vi "fmt_formatDataColumn.vi"(5 "styles map":string[](array[string]), 8 "error in (no error)":errorcluster, 9 "data":T1, 10 "channel index":i32, 11 "Format buffers in":T3) -> (0 "error out":errorcluster, 3 "Format buffers out":T3)   [LabVIEW 2017, in "NI_ExcelFile.lvlib"]
uses:
  <vilib>/express/express shared/NI_ExcelFile/NI_ExcelFile.lvlib
  <vilib>/express/express shared/NI_ExcelFile/Ctrls/fmt_formatBuffer.ctl
  <vilib>/express/express shared/NI_ExcelFile/Ctrls/TimeColumnMode.ctl
  <vilib>/express/express shared/NI_ExcelFile/Ctrls/Columns.ctl
  <vilib>/express/express shared/NI_ExcelFile/Ctrls/ColumnInfo.ctl
  <vilib>/express/express shared/NI_ExcelFile/Ctrls/DataType.ctl
  <vilib>/express/express shared/NI_ExcelFile/Ctrls/data_AllTypeData.ctl
  <vilib>/express/express shared/NI_ExcelFile/SubVIs/fmt_formatSingleCell (Numeric).vi
  <vilib>/express/express shared/NI_ExcelFile/SubVIs/fmt_timestampToExcel.vi
  <vilib>/express/express shared/NI_ExcelFile/SubVIs/fmt_formatSingleCell (String).vi
  <vilib>/express/express shared/NI_ExcelFile/SubVIs/fmt_escapeXML.vi
  <vilib>/express/express shared/NI_ExcelFile/SubVIs/fmt_getUTF-8Text.vi
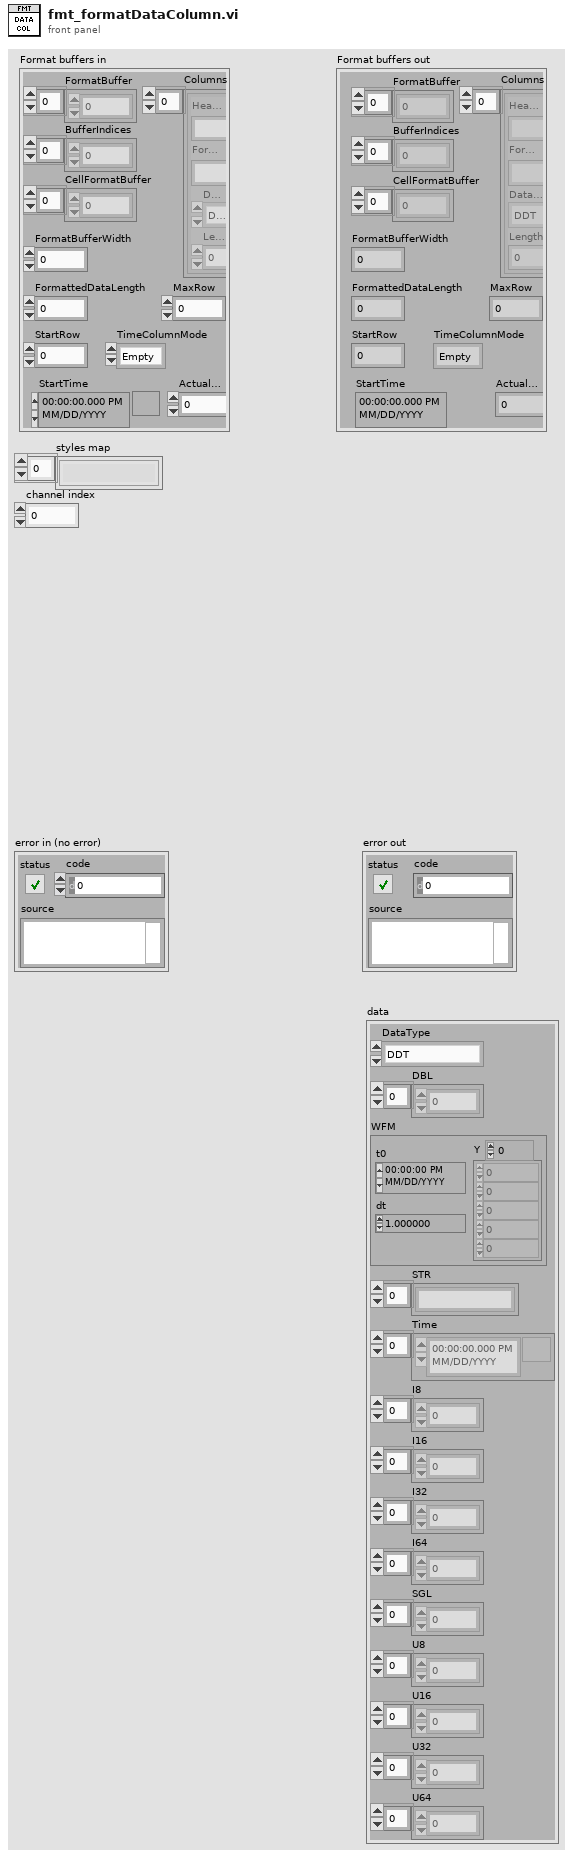
[diagram p1: front panel]
types:
  T1 = typedef "NI_ExcelFile.lvlib/data_AllTypeData.ctl" = cluster{"DataType":T2, "DBL":dbl[], "WFM":waveform(dbl), "STR":string[], "Time":timestamp[], "I8":i8[], "I16":i16[], "I32":i32[], "I64":i64[], "SGL":sgl[], "U8":u8[], "U16":u16[], "U32":u32[], "U64":u64[]}
  T2 = typedef "NI_ExcelFile.lvlib/DataType.ctl" = enum16{"DDT", "WFM", "Array of STR", "Array of DBL", "Array of I8", "Array of I16", "Array of I32", "Array of I64", "Array of SGL", "Array of U8", "Array of U16", "Array of U32", "Array of U64", "Array of Time"}
  T3 = typedef "NI_ExcelFile.lvlib/fmt_formatBuffer.ctl" = cluster{"FormatBuffer":u8[], "BufferIndices":i32[], "CellFormatBuffer":u8[], "FormatBufferWidth":i32, "FormattedDataLength":i32, "MaxRow":i32, "StartRow":i32, "TimeColumnMode":T4, "StartTime":timestamp, "Columns":T5, "ActualLength":i32}
  T4 = typedef "NI_ExcelFile.lvlib/TimeColumnMode.ctl" = enum16{"Empty", "OnePerCh", "One"}
  T5 = typedef "NI_ExcelFile.lvlib/Columns.ctl" = T6[]
  T6 = typedef "NI_ExcelFile.lvlib/ColumnInfo.ctl" = cluster{"Header":string, "Format":string, "DataType":T2, "Length":u64}
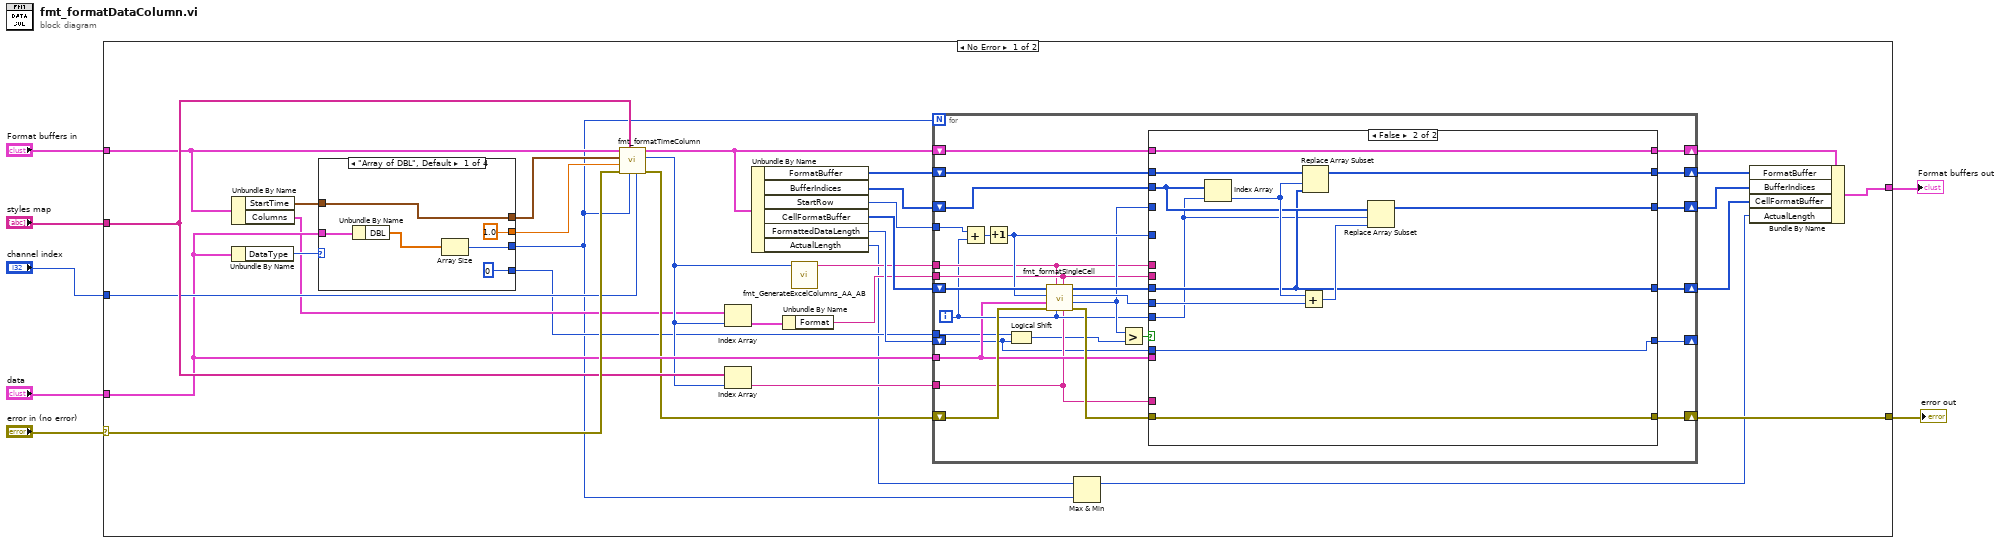
[diagram p0: block diagram]
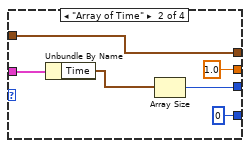
[diagram p2: hidden frame]
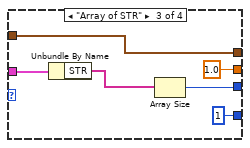
[diagram p3: hidden frame]
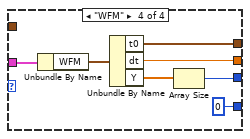
[diagram p4: hidden frame]
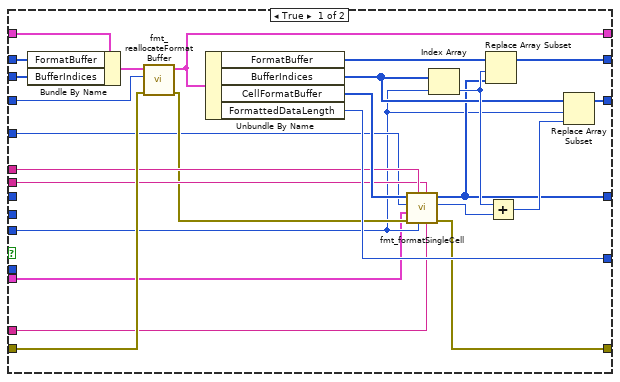
[diagram p5: hidden frame]
diagram:
  n1 = case shown="No Error" "error in (no error)" {
    selector: "error in (no error)" -> [w38 w130]
    tunnel: [w39 w129] -> w7
    tunnel: "styles map" -> [w36 _]
    tunnel: "channel index" -> [w35 _]
    tunnel: "Format buffers in" -> [w34 w129]
    tunnel: [w37 w130] -> w3
    tunnel: "data" -> [w33 _]
    frame No Error {
      n2 = Unbundle By Name(w34) -> ("StartTime"=w15:timestamp, "Columns"=w12:T5)
      n3 = Unbundle By Name(w33) -> ("DataType"=w16:T2)
      n4 = case shown="\"Array of DBL\", Default" w16 {
        tunnel: w15 -> [w45 w51 w57 _]
        tunnel: [w45 w51 w57 w62] -> w14
        tunnel: w33 -> [w43 w49 w55 w64]
        tunnel: [1.0 ("dt") 1.0 ("dt") 1.0 ("dt") w61] -> w13
        tunnel: [w42 w48 w54 w59] -> w9
        tunnel: [0 0 1 0] -> w11
        frame "Array of DBL", Default {
          n5 = Unbundle By Name(w43) -> ("DBL"=w41:dbl[])
          n6 = Array Size(array=w41) -> (size(s)=w42:i32)
        }
        frame "Array of Time" {
          n7 = Unbundle By Name(w49) -> ("Time"=w47:timestamp[])
          n8 = Array Size(array=w47) -> (size(s)=w48:i32)
        }
        frame "Array of STR" {
          n9 = Unbundle By Name(w55) -> ("STR"=w53:string[])
          n10 = Array Size(array=w53) -> (size(s)=w54:i32)
        }
        frame "WFM" {
          n11 = Unbundle By Name(w64) -> ("WFM"=w63:waveform(dbl))
          n12 = Unbundle By Name(w63) -> ("t0"=w62:timestamp, "dt"=w61:dbl, "Y"=w60:dbl[])
          n13 = Array Size(array=w60) -> (size(s)=w59:i32)
        }
      }
      n14 = call <vilib>:"fmt_formatTimeColumn.vi"("channel index"=w35, "length"=w9, "styles map"=w36, "error in (no error)"=w38, "dt"=w13, "t0"=w14, "format buffers in"=w34) -> ("error out"=w28:errorcluster, "data column index"=w18:i32, "format buffers out"=w27:T3)  [unwired: 2 in]
      n15 = Index Array(array=w12, index=w18) -> (element=w21:T6)
      n16 = Index Array(array=w36, index=w18) -> (element=w17:string)
      n17 = Unbundle By Name(w27) -> ("FormatBuffer"=w26:u8[], "BufferIndices"=w25:i32[], "StartRow"=w24:i32, "CellFormatBuffer"=w23:u8[], "FormattedDataLength"=w22:i32, "ActualLength"=w10:i32)
      n18 = Unbundle By Name(w21) -> ("Format"=w19:string)
      n19 = call <vilib>:"fmt_GenerateExcelColumns_AA_AB.vi"("NumColumns"=w18) -> ("Column"=w20:string)  [unwired: 10 in]
      n20 = for {
        N: w9 -> [_]
        shift-right: [w90] -> w31
        shift-left: w26 -> [w91]
        shift-right: [w88] -> w30
        shift-left: w25 -> [w89]
        shift-right: [w84] -> w29
        shift-left: w23 -> [w76]
        shift-right: [w83] -> w37
        shift-left: w28 -> [w79]
        shift-right: [w81] -> _
        shift-left: w22 -> [w65]
        shift-right: [w85] -> w32
        shift-left: w27 -> [w86]
        tunnel: w20 -> [w71]
        tunnel: w24 -> [w80]
        tunnel: w19 -> [w72]
        tunnel: w33 -> [w69]
        tunnel: w17 -> [w68]
        tunnel: w11 -> [w66]
        i -> [w70]
        n21 = Add(x=w80, y=w70) -> (x+y=w82:i32)
        n22 = Increment(x=w82) -> (x+1=w75:i32)
        n23 = Logical Shift(y=w66, x=w65) -> (x << y=w67:i32)
        n24 = call <vilib>:"fmt_formatSingleCell.vi"("style"=w68, "format string"=w72, "index"=w70, "column"=w71, "error in (no error)"=w79, "data"=w69, "row"=w75, "Format buffer"=w76) -> ("error out"=w78:errorcluster, "Formatted data length"=w73:i32, "Buffer size"=w74:i32, "Formatted buffer"=w77:u8[])
        n25 = Greater?(x=w73, y=w67) -> (0:w87:bool)
        n26 = case shown="False" w87 {
          tunnel: w91 -> [w115 w128]
          tunnel: w74 -> [_ w127]
          tunnel: [w109 w126] -> w90
          tunnel: w89 -> [w113 w122]
          tunnel: [w107 w124] -> w88
          tunnel: w77 -> [_ w120]
          tunnel: w86 -> [w116 w121]
          tunnel: [w106 w121] -> w85
          tunnel: w73 -> [w105 _]
          tunnel: [w101 w120] -> w84
          tunnel: w75 -> [w96 _]
          tunnel: w78 -> [w104 w119]
          tunnel: [w97 w119] -> w83
          tunnel: [w103 w118] -> w81
          tunnel: w65 -> [_ w118]
          tunnel: w70 -> [w94 w117]
          tunnel: w71 -> [w100 _]
          tunnel: w72 -> [w99 _]
          tunnel: w69 -> [w93 _]
          tunnel: w68 -> [w95 _]
          frame True {
            n27 = Bundle By Name(cluster=w116, "FormatBuffer"=w115, "BufferIndices"=w113) -> (w114:T3)
            n28 = call <vilib>:"fmt_reallocateFormatBuffer.vi"("error in (no error)"=w104, "Formatted data length"=w105, "Format buffers in"=w114) -> ("error out"=w98:errorcluster, "Format buffers out"=w106:T3)  [unwired: 7 in]
            n29 = Unbundle By Name(w106) -> ("FormatBuffer"=w110:u8[], "BufferIndices"=w108:i32[], "CellFormatBuffer"=w102:u8[], "FormattedDataLength"=w103:i32)
            n30 = call <vilib>:"fmt_formatSingleCell.vi"("style"=w95, "format string"=w99, "index"=w94, "column"=w100, "error in (no error)"=w98, "data"=w93, "row"=w96, "Format buffer"=w102) -> ("error out"=w97:errorcluster, "Buffer size"=w92:i32, "Formatted buffer"=w101:u8[])  [unwired: 1 out]
            n31 = Index Array(array=w108, index=w94) -> (element=w111:i32)
            n32 = Replace Array Subset(array=w110, new element=w101, index=w111) -> (w109:u8[])
            n33 = Add(x=w111, y=w92) -> (x+y=w112:i32)
            n34 = Replace Array Subset(array=w108, new element=w112, index=w94) -> (w107:i32[])
          }
          frame False {
            n35 = Index Array(array=w122, index=w117) -> (element=w123:i32)
            n36 = Add(x=w123, y=w127) -> (x+y=w125:i32)
            n37 = Replace Array Subset(array=w128, new element=w120, index=w123) -> (w126:u8[])
            n38 = Replace Array Subset(array=w122, new element=w125, index=w117) -> (w124:i32[])
          }
        }
      }
      n39 = Max & Min(x=w10, y=w9) -> (max(x,y)=w8:i32)  [unwired: 1 out]
      n40 = Bundle By Name(cluster=w32, "FormatBuffer"=w31, "BufferIndices"=w30, "CellFormatBuffer"=w29, "ActualLength"=w8) -> (w39:T3)
    }
    frame Error {
    }
  }
  "Format buffers out" <- w7
  "error out" <- w3
